vi "AIT 1553 - Create BM Sysdef Tree Messages.vi"(7 "Called From SysDef API (F)":bool, 8 "error in":errorcluster, 9 "BM Messages":T1[](array[typedef]), 10 "Section Ptr":T3 format="%.0x") -> (0 "error out":errorcluster)   [LabVIEW 2013, in "AIT 1553 Custom Device.lvlib"]
uses:
  AIT 1553 Custom Device.lvlib
  <vilib>/NI Veristand/Custom Device API/Custom Device Item Ref.ctl
  Controls/1553_BM_Message.ctl
  Controls/1553 Param.ctl
  <vilib>/NI Veristand/Custom Device API/Custom Device Channel Type.ctl
  <vilib>/NI Veristand/Custom Device API/Custom Device Channel.ctl
  Controls and Global/Global.vi
  <vilib>/NI Veristand/Custom Device API/Custom Device API.lvlib
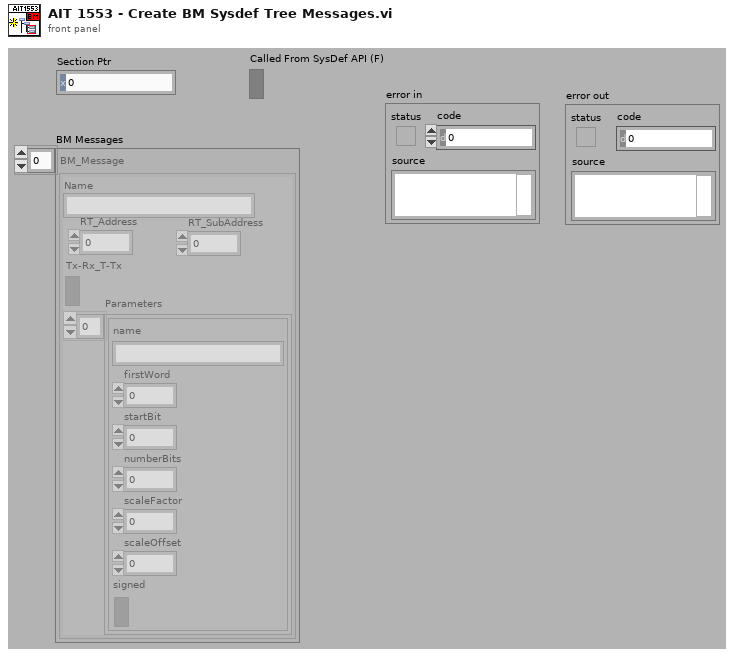
[diagram p1: front panel]
types:
  T1 = typedef "AIT 1553 Custom Device.lvlib/1553_BM_Message.ctl" = cluster{"RT_Address":u8, "RT_SubAddress":u8, "Tx-Rx_T-Tx":bool, "Parameters":T2[], "Name":string}
  T2 = typedef "AIT 1553 Custom Device.lvlib/1553 Param.ctl" = cluster{"name":string, "firstWord":i32, "startBit":i32, "numberBits":i32, "scaleFactor":dbl, "scaleOffset":dbl, "signed":bool}
  T3 = typedef "Custom Device API.lvlib/Custom Device Item Ref.ctl" = u64
  T4 = typedef "Custom Device API.lvlib/Custom Device Channel.ctl" = cluster{"Type":T5, "Units":string, "Default Value":dbl, "Faultable":bool, "Scalable":bool}
  T5 = typedef "Custom Device API.lvlib/Custom Device Channel Type.ctl" = enum16{"Input", "Output"}
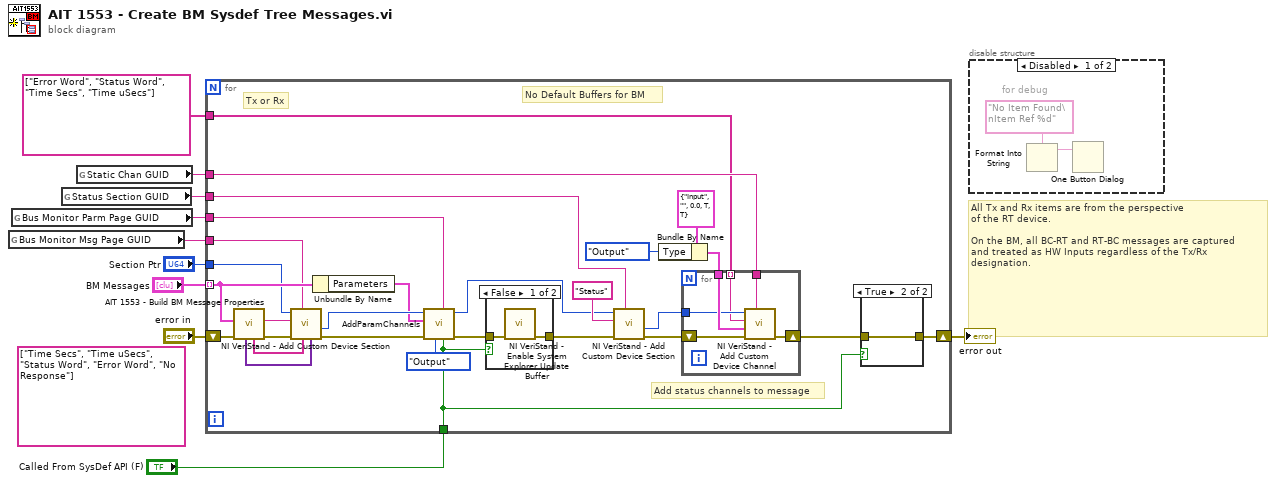
[diagram p0: block diagram]
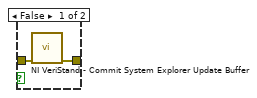
[diagram p3: hidden frame]
diagram:
  (unwired) string[] ["Time Secs", "Time uSecs", "Status Word", "Error Word", "No Response"]
  # "All Tx and Rx items are from the perspective \nof the RT device.\n\nOn the BM, all BC-RT and RT-BC messages are captured\nand treated as HW Inputs regardless of the Tx/Rx \ndesignation."
  n1 = global read "Global.vi" "Bus Monitor Msg Page GUID"() -> (w7:string)
  n2 = global read "Global.vi" "Bus Monitor Parm Page GUID"() -> (w5:string)
  n3 = global read "Global.vi" "Status Section GUID"() -> (w3:string)
  n4 = global read "Global.vi" "Static Chan GUID"() -> (w4:string)
  n5 = for {
    shift-right: [w13] -> w10
    shift-left: "error in" -> [w34]
    tunnel: "Section Ptr" -> [w29]
    tunnel: "BM Messages" -> [w31] mode=indexing
    tunnel: w7 -> [w30]
    tunnel: w5 -> [w28]
    tunnel: w4 -> [w26]
    tunnel: w3 -> [w17]
    tunnel: string[] ["Error Word", "Status Word", "Time Secs", "Time uSecs"] -> [w25]
    tunnel: "Called From SysDef API (F)" -> [w12]
    # "Add status channels to message"
    # "Tx or Rx"
    # "No Default Buffers for BM"
    n6 = call "AIT 1553 - Build BM Message Properties.vi"("error in (no error)"=w34, "BM_Message"=w31) -> ("error out"=w36:errorcluster, "name"=w35:string, "Prop Names"=w37:string[], "Prop Values"=w38:variant[])  [unwired: 5 in, 1 out]
    n7 = call <vilib>:"NI VeriStand - Add Custom Device Section.vi"("Property Values"=w38, "Property names"=w37, "GUID (Default Section)"=w30, "error in (no error)"=w36, "Section Name"=w35, "Parent Ref in"=w29) -> ("error out"=w32:errorcluster, "Section Ptr"=w33:T3)  [unwired: 2 in, 2 out]
    n8 = Unbundle By Name(w31) -> ("Parameters"=w24:T2[])
    n9 = call "AddParamChannels.vi"("Called From SysDef API (F)"=w12, "Parm Page GUID"=w28, "Type"=Custom_Device_Channel_Type."Output", "error in"=w32, "Parameters to add"=w24, "Node Ref In"=w33) -> ("error out"=w15:errorcluster, "Node Ref Out"=w16:T3)  [unwired: 4 in]
    n10 = case shown="False" w12 {
      tunnel: w15 -> [w43 w44]
      tunnel: [w42 w44] -> w14
      frame False {
        n11 = call <vilib>:"NI VeriStand - Enable System Explorer Update Buffer.vi"("error in (no error)"=w43) -> ("error out"=w42:errorcluster)  [unwired: 10 in]
      }
      frame True {
      }
    }
    n12 = call <vilib>:"NI VeriStand - Add Custom Device Section.vi"("GUID (Default Section)"=w17, "error in (no error)"=w14, "Section Name"="Status", "Parent Ref in"=w16) -> ("error out"=w21:errorcluster, "Section Ptr"=w22:T3)  [unwired: 4 in, 2 out]
    n13 = Bundle By Name(cluster=T4 {"Type"=enum."Input", "Units"="", "Default Value"=0.0, "Faultable"=TRUE, "Scalable"=TRUE} ("Channel"), "Type"=Custom_Device_Channel_Type."Output") -> (w20:T4)
    n14 = for {
      tunnel: w20 -> [w49]
      tunnel: w26 -> [w48]
      tunnel: w22 -> [w46]
      tunnel: w25 -> [w45] mode=indexing
      shift-right: [w50] -> w11
      shift-left: w21 -> [w47]
      n15 = call <vilib>:"NI VeriStand - Add Custom Device Channel.vi"("GUID (Default Channel)"=w48, "error in (no error)"=w47, "Channel"=w49, "Channel Name"=w45, "Parent Ref in"=w46) -> ("error out"=w50:errorcluster)  [unwired: 3 in, 3 out]
    }
    n16 = case shown="True" w12 {
      tunnel: w11 -> [w40 w41]
      tunnel: [w39 w41] -> w13
      frame False {
        n17 = call <vilib>:"NI VeriStand - Commit System Explorer Update Buffer.vi"("error in (no error)"=w40) -> ("error out"=w39:errorcluster)  [unwired: 10 in]
      }
      frame True {
      }
    }
  }
  "error out" <- w10
  n18 = disable-structure shown="Disabled" {
    frame Disabled {
      # "for debug"
      n19 = Format Into String(format string="No Item Found\nItem Ref %d" ("message")) -> (resulting string=w53:string, w51:T3)  [unwired: 2 in, 1 out]
      n20 = One Button Dialog(message=w53) -> (true=w54:bool)  [unwired: 1 in]
    }
    frame Enabled {
    }
  }
